vi "AssignAndCount60_tester.vi"(0 "Photon counter area 1 in":u16, 5 "Photon counter area 2 in":u16, 7 "Laser bits in":bool[](array[boolean])=[FALSE, FALSE, FALSE, FALSE, FALSE, FALSE, FALSE, FALSE, FALSE, FALSE, FALSE, FALSE, FALSE, FALSE, FALSE, FALSE, FALSE, FALSE, FALSE, FALSE, FALSE, FALSE, FALSE, FALSE, FALSE, FALSE, FALSE, FALSE, FALSE, FALSE, FALSE, FALSE, FALSE, FALSE, FALSE, FALSE, FALSE, FALSE, FALSE, FALSE, FALSE, FALSE, FALSE, FALSE, FALSE, FALSE, FALSE, FALSE, FALSE, FALSE, FALSE, FALSE, FALSE, FALSE, FALSE, FALSE, FALSE, FALSE, FALSE, FALSE], 9 "PMT bits in":bool[](array[boolean])=[FALSE, FALSE, FALSE, FALSE, FALSE, FALSE, FALSE, FALSE, FALSE, FALSE, FALSE, FALSE, FALSE, FALSE, FALSE, FALSE, FALSE, FALSE, FALSE, FALSE, FALSE, FALSE, FALSE, FALSE, FALSE, FALSE, FALSE, FALSE, FALSE, FALSE, FALSE, FALSE, FALSE, FALSE, FALSE, FALSE, FALSE, FALSE, FALSE, FALSE, FALSE, FALSE, FALSE, FALSE, FALSE, FALSE, FALSE, FALSE, FALSE, FALSE, FALSE, FALSE, FALSE, FALSE, FALSE, FALSE, FALSE, FALSE, FALSE, FALSE], 11 "Last laser bit in":bool, 12 "Last region":bool=TRUE) -> (4 "Photon counter area 1 out":u16, 6 "Photon counter area 2 out":u16, 8 "Region array out":bool[](array[boolean]), 14 "New last region out":bool, 15 "New last laser bit out":bool)   [LabVIEW 2012]
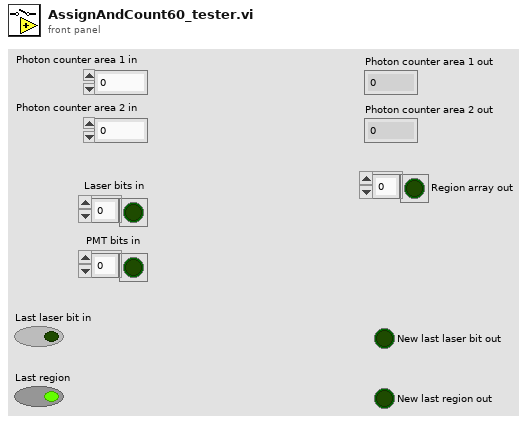
[diagram p1: front panel]
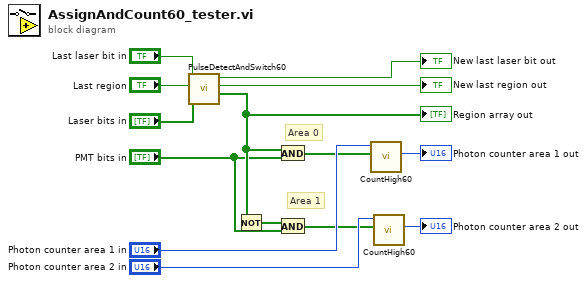
[diagram p0: block diagram]
diagram:
  # "Area 1"
  # "Area 0"
  n1 = call "PulseDetectAndSwitch60.vi"("Laser bits in"="Laser bits in", "Last region"="Last region", "Last laser bit in"="Last laser bit in") -> ("Region array out"=w13:bool[], "New last region out"=→"New last region out":bool, "New last laser bit out"=→"New last laser bit out":bool)  [unwired: 6 in]
  "Region array out" <- w13
  n2 = Not(x=w13) -> (.not. x?=w12:bool[])
  n3 = And(x=w13, y="PMT bits in") -> (x .and. y?=w5:bool[])
  n4 = And(x=w12, y="PMT bits in") -> (x .and. y?=w2:bool[])
  n5 = call "CountHigh60.vi"("60bit input"=w5, "Previous high count"="Photon counter area 1 in") -> ("New high count"=→"Photon counter area 1 out":u16)  [unwired: 9 in]
  n6 = call "CountHigh60.vi"("60bit input"=w2, "Previous high count"="Photon counter area 2 in") -> ("New high count"=→"Photon counter area 2 out":u16)  [unwired: 9 in]
